vi "new OR Filter.vi"(5 "a":refnum<class "Filter.lvclass">, 9 "b":refnum<class "Filter.lvclass">) -> (8 "a or b":refnum<class "Filter.lvclass">)   [LabVIEW 2016, in "OR Filter.lvclass"]
uses:
  OR Filter.lvclass
  Filter Parent/Filter.lvclass
  C:/github/VeriStand-FPGA-Resource-Manager/Source/Client/Test CD/FPGA RM Test Client/Source/System Explorer/Filters/Filter Parent/Filter.lvclass
  OR Filter.lvclass/OR Filter.ctl
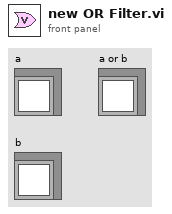
[diagram p1: front panel]
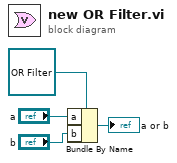
[diagram p0: block diagram]
diagram:
  n1 = Bundle By Name(cluster=refnum<class "OR Filter.lvclass"> refnum ("OR Filter in"), "a"="a", "b"="b") -> (→"a or b":refnum<class "OR Filter.lvclass">)
